vi "散斑图像作用结果累加.vi"(1 "图像连接一维数组":dbl[](array[numeric]), 2 "散斑行数":i32, 3 "散斑二维数组":dbl[][](array[numeric])) -> (0 "散斑图像作用结果求和":dbl)   [LabVIEW 2018]
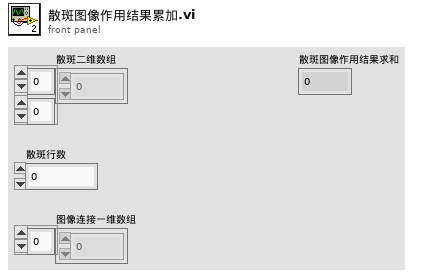
[diagram p1: front panel]
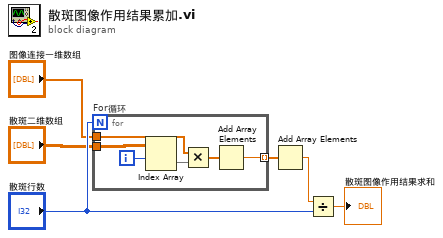
[diagram p0: block diagram]
diagram:
  n1 = for "For循环" {
    N: "散斑行数" -> [_]
    tunnel: "散斑二维数组" -> [w12]
    tunnel: "图像连接一维数组" -> [w8]
    tunnel: [w9] -> w6 mode=indexing
    i -> [w11]
    n2 = Index Array(array=w12, index (row)=w11) -> (element=w7:dbl[])  [unwired: 1 in]
    n3 = Multiply(x=w8, y=w7) -> (x*y=w10:dbl[])
    n4 = Add Array Elements(numeric array=w10) -> (sum=w9:dbl)
  }
  n5 = Add Array Elements(numeric array=w6) -> (sum=w5:dbl)
  n6 = Divide(x=w5, y="散斑行数") -> (x/y=→"散斑图像作用结果求和":dbl)
